vi "icListen 1 Enabled.vi"() -> ()   [LabVIEW 2020, in "PAM Library.lvlib"]
uses:
  PAM Library.lvlib
panel:
  in  "icListen 1 Enabled":bool
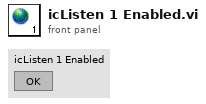
[diagram p1: front panel]
diagram:
